vi "Case Control.vi"(5 "Range 80%":dbl, 7 "Range 60%":dbl, 8 "error in":errorcluster, 10 "BPM input":dbl, 11 "Arduino Resource":T1={"VISA resource"="", "Board Type"=enum."Uno", "Connection Type"=enum."USB / Serial", "Bytes Per Packet (15)"=15}) -> (0 "error out":errorcluster)   [LabVIEW 2016]
uses:
  <vilib>/LabVIEW Interface for Arduino/Type Defs/Arduino Resource.ctl
  <vilib>/LabVIEW Interface for Arduino/Type Defs/Board Type.ctl
  <vilib>/LabVIEW Interface for Arduino/LabVIEW Interface for Arduino.lvlib
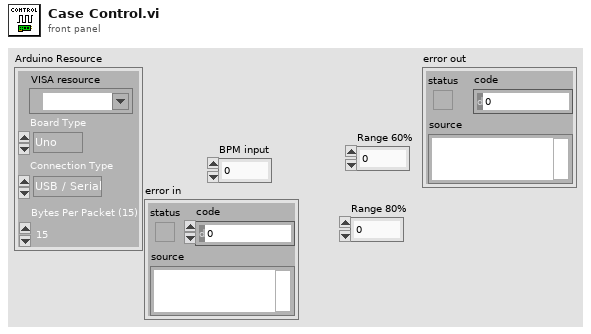
[diagram p1: front panel]
types:
  T1 = typedef "LabVIEW Interface for Arduino.lvlib/Arduino Resource.ctl" = cluster{"VISA resource":refnum<visa-resource-name>, "Board Type":T2, "Connection Type":enum8{"USB / Serial"}, "Bytes Per Packet (15)":u8}
  T2 = typedef "LabVIEW Interface for Arduino.lvlib/Board Type.ctl" = enum16{"Uno", "Dimuelanove w/Atmega 328", "Mega 2560"}
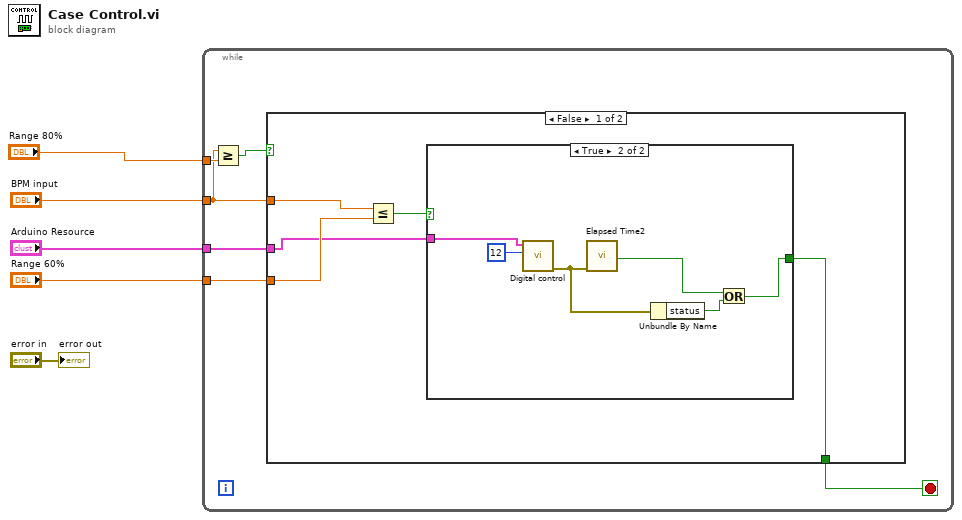
[diagram p0: block diagram]
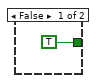
[diagram p2: hidden frame]
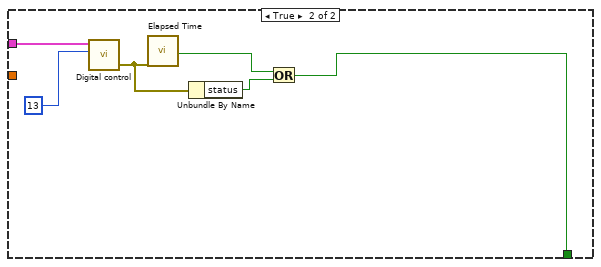
[diagram p3: hidden frame]
diagram:
  n1 = while {
    tunnel: "Range 80%" -> [w11]
    tunnel: "BPM input" -> [w7]
    tunnel: "Arduino Resource" -> [w9]
    tunnel: "Range 60%" -> [w6]
    stop <- w8 stop-if-true
    n2 = Greater Or Equal?(x=w7, y=w11) -> (x >= y?=w10:bool)
    n3 = case shown="False" w10 {
      tunnel: w9 -> [w12 w28]
      tunnel: [w13 w24] -> w8
      tunnel: w7 -> [w16 _]
      tunnel: w6 -> [w15 _]
      frame False {
        n4 = Less Or Equal?(x=w16, y=w15) -> (x <= y?=w14:bool)
        n5 = case shown="True" w14 {
          tunnel: [TRUE ("Time has Elapsed") w18] -> w13
          tunnel: w12 -> [_ w22]
          frame False {
          }
          frame True {
            n6 = call "Digital control.vi"("Digital I/O Pin (0)"=u8 12, "Arduino Resource"=w22) -> ("error out"=w20:errorcluster)  [unwired: 8 in, 1 out]
            n7 = call "Elapsed Time2"("error in (no error)"=w20) -> ("Time has Elapsed"=w19:bool)  [unwired: 11 in, 7 out]
            n8 = Unbundle By Name(w20) -> ("status"=w21:bool)
            n9 = Or(x=w19, y=w21) -> (x .or. y?=w18:bool)
          }
        }
      }
      frame True {
        n10 = call "Digital control.vi"("Digital I/O Pin (0)"=u8 13, "Arduino Resource"=w28) -> ("error out"=w27:errorcluster)  [unwired: 8 in, 1 out]
        n11 = call "Elapsed Time"("error in (no error)"=w27) -> ("Time has Elapsed"=w25:bool)  [unwired: 11 in, 7 out]
        n12 = Unbundle By Name(w27) -> ("status"=w26:bool)
        n13 = Or(x=w25, y=w26) -> (x .or. y?=w24:bool)
      }
    }
  }
  "error out" <- "error in"
